vi "Ouit_Name.vi"(8 "error in (no error)":errorcluster, 9 "BL":bool, 10 "OutPut":T1, 11 "FlowCtrl in":refnum<class "Station Action.lvclass">) -> (0 "error out":errorcluster, 3 "FlowCtrl out":refnum<class "Station Action.lvclass">)   [LabVIEW 2019]
uses:
  Station Action.lvclass
  FlowCtrl Class/Ctrl/Auto Inspection_Out Name.ctl
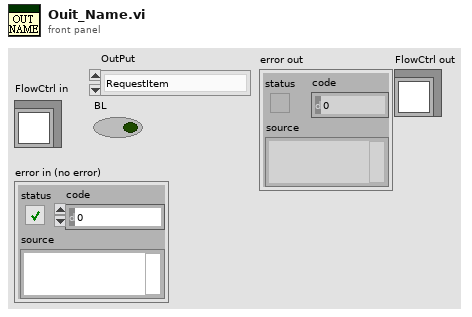
[diagram p1: front panel]
types:
  T1 = typedef "Auto Inspection_Out Name.ctl" = enum16{"RequestItem", "ConeyorMotor", "WorkPosStopper", "SlowConveyor", "Rise", "Fix", "ImformOut"}
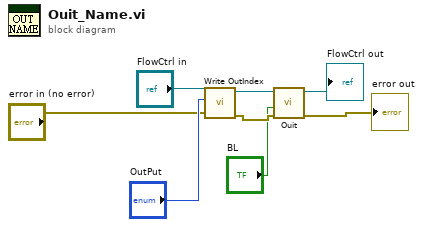
[diagram p0: block diagram]
diagram:
  n1 = call-dynamic "Write OutIndex.vi"("error in (no error)"="error in (no error)", "OutIndex"="OutPut", "Station Action in"="FlowCtrl in") -> ("error out"=w5:errorcluster, "Station Action out"=w3:refnum<class "Station Action.lvclass">)  [unwired: 7 in]
  n2 = call-dynamic "Ouit.vi"("error in (no error)"=w5, "BL"="BL", "FlowCtrl in"=w3) -> ("error out"=→"error out":errorcluster, "FlowCtrl out"=→"FlowCtrl out":refnum<class "Station Action.lvclass">)  [unwired: 7 in]
